vi "LaserLineDetection_Intensity_IntensityCheck.vi"(8 "Yarray":i32[](array[numeric]), 9 "I_AVERAGEarray":u8[](array[numeric]), 10 "INTENSITYarray":u8[](array[numeric]), 11 "Least Square Accepted":bool) -> (3 "Sampled Search Accepted":bool)   [LabVIEW 2013]
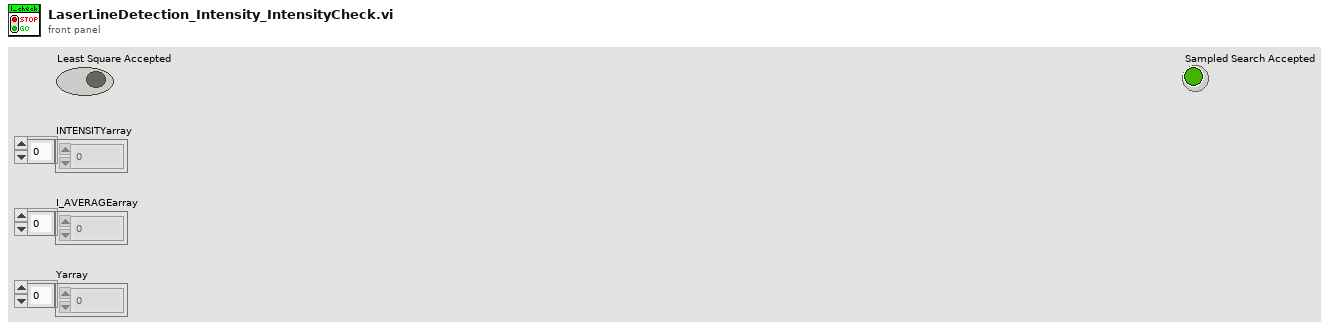
[diagram p1: front panel]
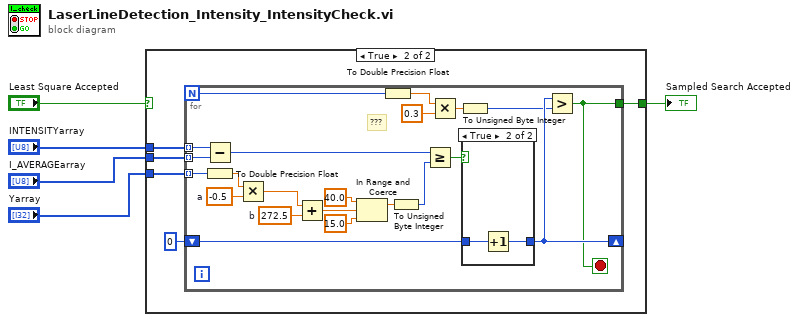
[diagram p0: block diagram]
diagram:
  n1 = case shown="True" "Least Square Accepted" {
    selector: "Least Square Accepted" -> [w6 _]
    tunnel: [w6 w8] -> w3
    tunnel: "INTENSITYarray" -> [_ w9]
    tunnel: "I_AVERAGEarray" -> [_ w11]
    tunnel: "Yarray" -> [_ w7]
    frame False {
    }
    frame True {
      n2 = for {
        N -> [w28]
        tunnel: w9 -> [w33] mode=indexing
        tunnel: w11 -> [w32] mode=indexing
        shift-right: [w24] -> _
        shift-left: u8 0 ("x") -> [w29]
        tunnel: [w22] -> w8
        tunnel: w7 -> [w13] mode=indexing
        stop <- w22 stop-if-true
        w16 = 272.5  # b
        w14 = -0.5  # a
        # "???"
        n3 = Subtract(x=w33, y=w32) -> (x-y=w31:u8)
        n4 = To Double Precision Float(number=w13) -> (double precision float=w20:dbl)
        n5 = Multiply(x=w20, y=w14) -> (x*y=w15:dbl)
        n6 = Add(x=w15, y=w16) -> (x+y=w17:dbl)
        n7 = In Range and Coerce(upper limit=40.0, x=w17, lower limit=15.0) -> (coerced(x)=w21:dbl)  [unwired: 1 out]
        n8 = To Double Precision Float(number=w28) -> (double precision float=w27:dbl)
        n9 = To Unsigned Byte Integer(number=w21) -> (unsigned 8bit integer=w12:u8)
        n10 = Greater Or Equal?(x=w31, y=w12) -> (x >= y?=w30:bool)
        n11 = Multiply(x=w27, y=0.3) -> (x*y=w25:dbl)
        n12 = To Unsigned Byte Integer(number=w25) -> (unsigned 8bit integer=w23:u8)
        n13 = case shown="True" w30 {
          tunnel: w29 -> [w34 w36]
          tunnel: [w34 w35] -> w24
          frame False {
          }
          frame True {
            n14 = Increment(x=w36) -> (x+1=w35:u8)
          }
        }
        n15 = Greater?(x=w24, y=w23) -> (0:w22:bool)
      }
    }
  }
  "Sampled Search Accepted" <- w3
